vi "Distance tot Line.vi"(8 "B":dbl, 9 "M":dbl, 10 "Y":dbl, 11 "X":dbl) -> (2 "Distance":dbl)   [LabVIEW 2017]
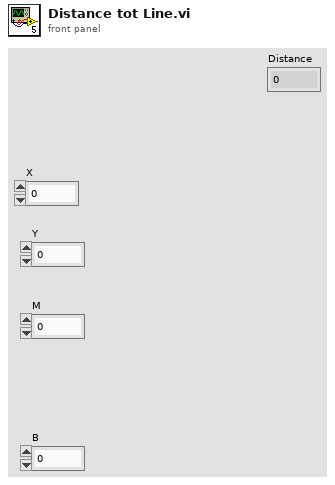
[diagram p1: front panel]
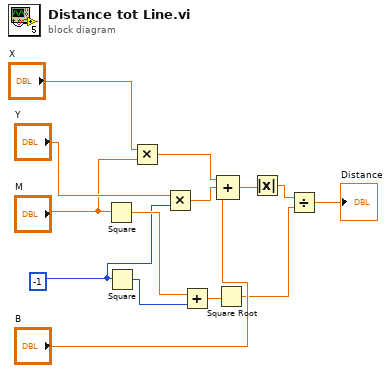
[diagram p0: block diagram]
diagram:
  w9 = -1
  n1 = Square(x="M") -> (x^2=w13:dbl)
  n2 = Square(x=w9) -> (x^2=w12:i32)
  n3 = Multiply(x="X", y="M") -> (x*y=w8:dbl)
  n4 = Multiply(x="Y", y=w9) -> (x*y=w6:dbl)
  n5 = Add(x=w13, y=w12) -> (x+y=w11:dbl)
  n6 = Square Root(x=w11) -> (sqrt(x)=w2:dbl)
  n7 = Compound Arithmetic op=ADD(w8, w6, "B") -> (w4:dbl)
  n8 = Absolute Value(x=w4) -> (abs(x)=w3:dbl)
  n9 = Divide(x=w3, y=w2) -> (x/y=→"Distance":dbl)
